vi "SubVI_curva_de_bezier.vi"(2 "Nº de divisões da curva de Bézier (padrão: 20 divisões = 21 pontos)":i32=20, 3 "número de pontos que a matriz deve retornar (padrão: nº de divisões + 1)":i64, 4 "String in":string) -> (0 "result string":string, 1 "matrix":T1)   [LabVIEW 2017]
uses:
  <vilib>/Analysis/Matrix/Datatypes/RealMatrix.ctl
  <vilib>/Analysis/Matrix/NI_Matrix.lvlib
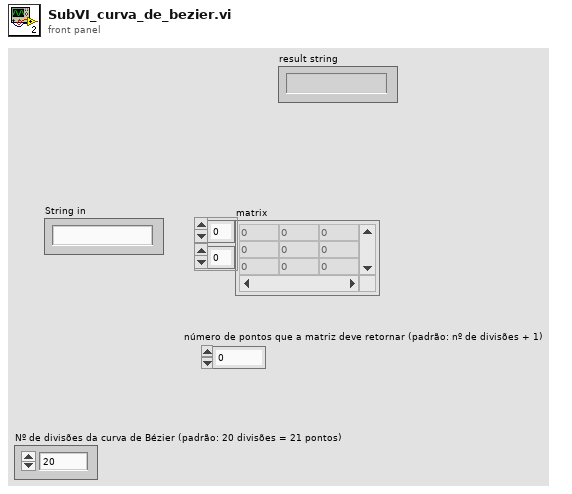
[diagram p1: front panel]
types:
  T1 = typedef "NI_Matrix.lvlib/RealMatrix.ctl" = dbl[][]
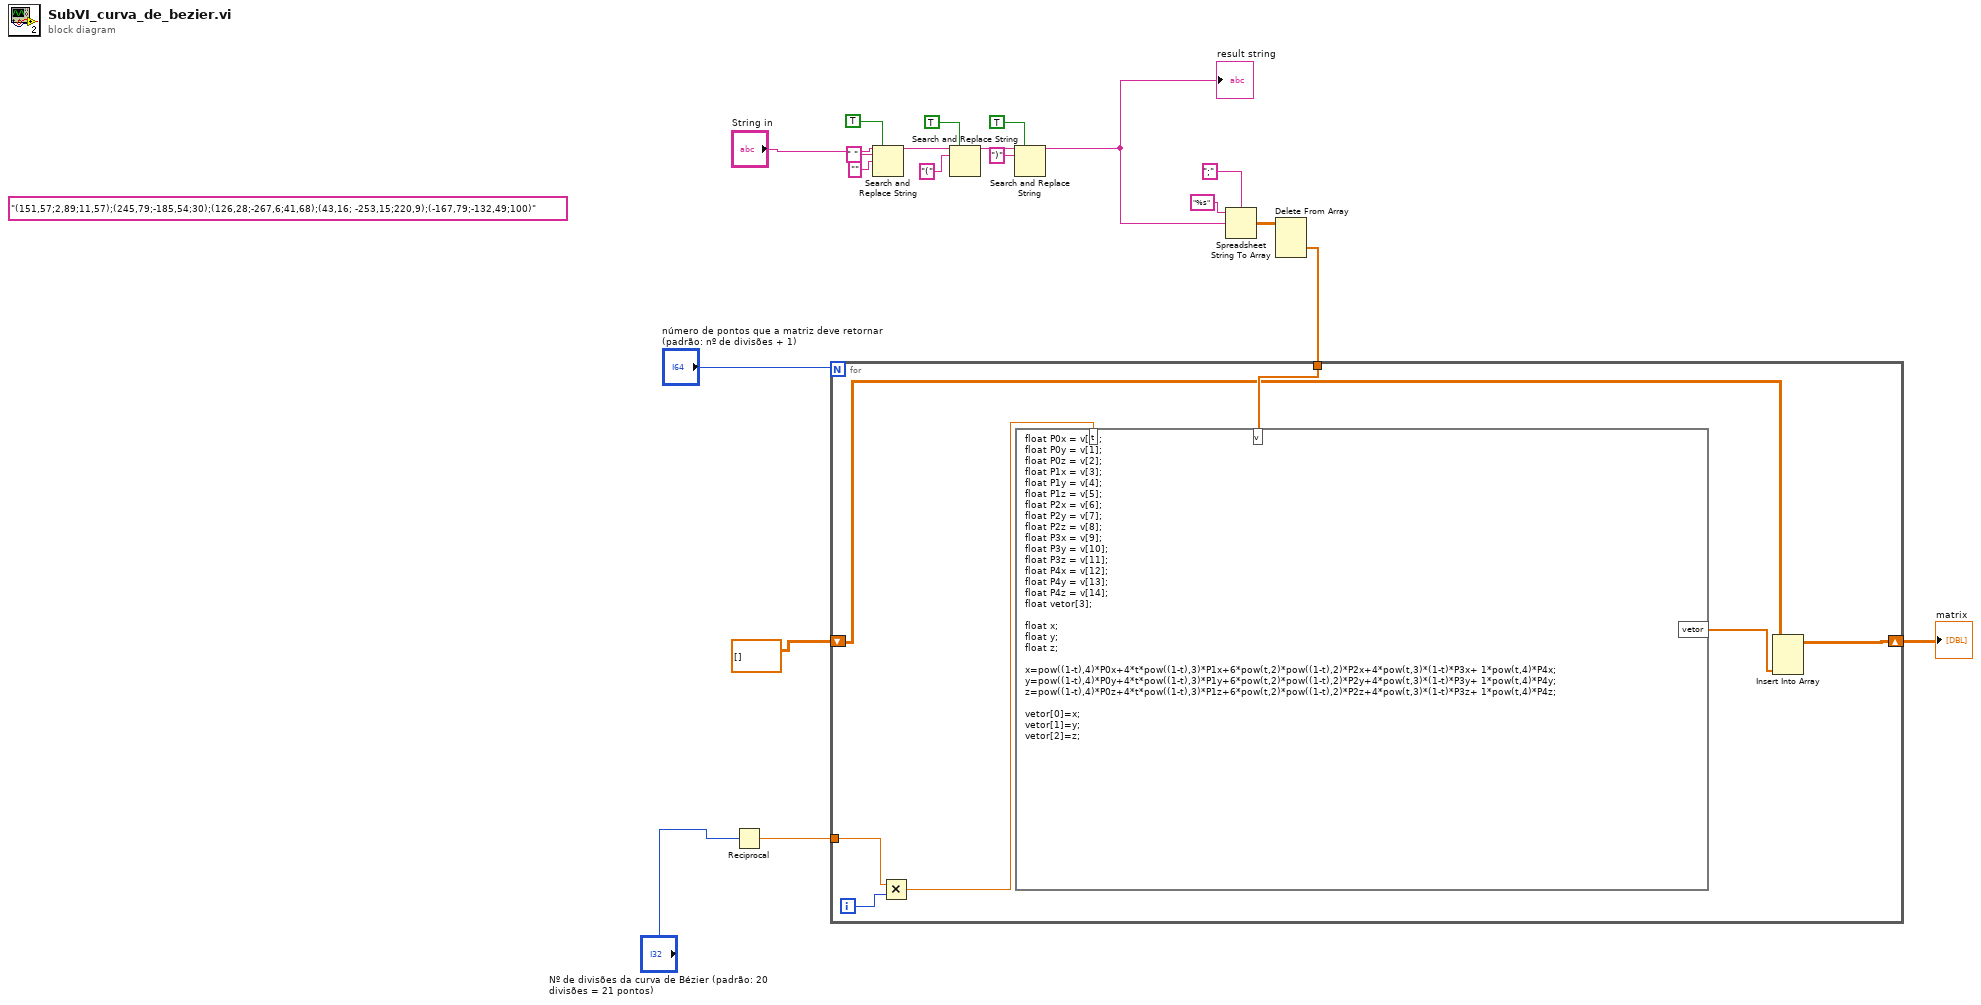
[diagram p0: block diagram]
diagram:
  (unwired) "(151,57;2,89;11,57);(245,79;-185,54;30);(126,28;-267,6;41,68);(43,16; -253,15;220,9);(-167,79;-132,49;100)" ("String 2")
  n1 = Reciprocal(x="Nº de divisões da curva de Bézier (padrão: 20 divisões = 21 pontos)") -> (1/x=w19:dbl)
  n2 = Search and Replace String(replace all?=TRUE ("replace all? (F)"), input string="String in", search string=" ", replace string="" ("replace string (\"\")")) -> (result string=w14:string)  [unwired: 4 in, 3 out]
  n3 = Search and Replace String(replace all?=TRUE ("replace all? (F)"), input string=w14, search string="(") -> (result string=w3:string)  [unwired: 5 in, 3 out]
  n4 = Search and Replace String(replace all?=TRUE ("replace all? (F)"), input string=w3, search string=")") -> (result string=w16:string)  [unwired: 5 in, 3 out]
  "result string" <- w16
  n5 = Spreadsheet String To Array(delimiter (Tab)=";", format string="%s", spreadsheet string=w16) -> (array=w8:dbl[][])  [unwired: 1 in]
  n6 = Delete From Array(array=w8) -> (deleted portion=w9:dbl[])  [unwired: 3 in, 1 out]
  n7 = for {
    N: "número de pontos que a matriz deve retornar (padrão: nº de divisões + 1)" -> [_]
    tunnel: w9 -> [w27]
    shift-right: [w22] -> w11
    shift-left: T1 [] ("matrix") -> [w25]
    tunnel: w19 -> [w21]
    i -> [w26]
    n8 = Multiply(x=w21, y=w26) -> (x*y=w23:dbl)
    n9 = formula code="float P0x = v[0];\nfloat P0y = v[1];\nfloat P0z = v[2];\nfloat P1x = v[3];\nfloat P1y = v[4];\nfloat P1z = v[5];\nfloat P2x = v[6];\nfloat P2y = v[7];\nfloat P2z = v[8];\nfloat P3x = v[9];\nfloat P3y = v[10];\nfloat P3z = v[11];\nfloat P4x = v[12];\nfloat P4y = v[13];\nfloat P4z = v[14];\nfloat vetor[3];\n\nfloat x;\nfloat y;\nfloat z;\n\nx=pow((1-t),4)*P0x+4*t*pow((1-t),3)*P1x+6*pow(t,2)*pow((1-t),2)*P2x+4*pow(t,3)*(1-t)*P3x+ 1*pow(t,4)*P4x;\ny=pow((1-t),4)*P0y+4*t*pow((1-t),3)*P1y+6*pow(t,2)*pow((1-t),2)*P2y+4*pow(t,3)*(1-t)*P3y+ 1*pow(t,4)*P4y;\nz=pow((1-t),4)*P0z+4*t*pow((1-t),3)*P1z+6*pow(t,2)*pow((1-t),2)*P2z+4*pow(t,3)*(1-t)*P3z+ 1*pow(t,4)*P4z;\n\nvetor[0]=x;\nvetor[1]=y;\nvetor[2]=z;"("v"=w27, "t"=w23) -> ("vetor"=w24:dbl[])
    n10 = Insert Into Array(array=w25, new element=w24) -> (w22:T1)  [unwired: 2 in]
  }
  "matrix" <- w11
